vi "Create Log File.vi"(8 "error in":errorcluster, 11 "Sys Log in":refnum<class "System Log.lvclass">) -> (0 "error out":errorcluster, 3 "Sys Log out":refnum<class "System Log.lvclass">)   [LabVIEW 2014, in "System Log.lvclass"]
uses:
  System Log.lvclass
  System Log.lvclass/System Log.ctl
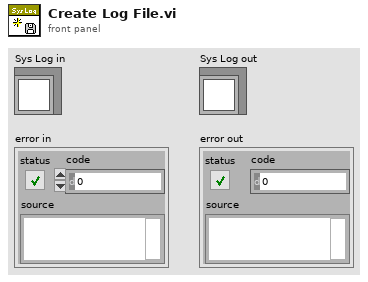
[diagram p1: front panel]
types:
  T1 = enum16{"open", "replace", "create", "open or create", "replace or create", "replace or create with confirmation"}
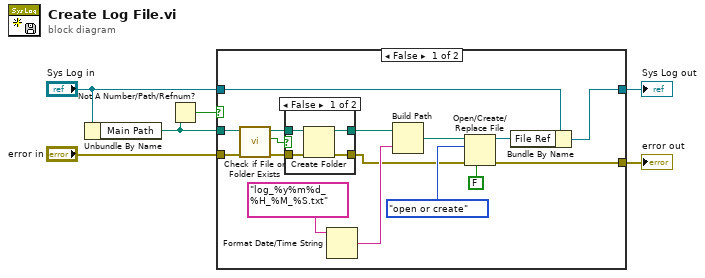
[diagram p0: block diagram]
diagram:
  n1 = Unbundle By Name("Sys Log in") -> ("Main Path"=w6:path)
  n2 = Not A Number/Path/Refnum?(number/path/refnum=w6) -> (NaN/Path/Refnum?=w1:bool)
  n3 = case shown="False" w1 {
    tunnel: "Sys Log in" -> [w22 w30]
    tunnel: [w21 w30] -> w3
    tunnel: "error in" -> [w15 w29]
    tunnel: [w19 w29] -> w5
    tunnel: w6 -> [w16 _]
    frame False {
      n4 = call <vilib>:"Check if File or Folder Exists.vi"("error in (no error)"=w15, "path"=w16) -> ("error out"=w12:errorcluster, "file or folder exists?"=w14:bool, "dup path"=w13:path)  [unwired: 7 in]
      n5 = case shown="False" w14 {
        tunnel: w13 -> [w26 w28]
        tunnel: w12 -> [w25 w27]
        tunnel: [w24 w28] -> w11
        tunnel: [w23 w27] -> w8
        frame False {
          n6 = Create Folder(path (use dialog)=w26, error in=w25) -> (created path=w24:path, error out=w23:errorcluster)  [unwired: 1 in, 1 out]
        }
        frame True {
        }
      }
      n7 = Format Date/Time String(time format string (%c)="log_%y%m%d_%H_%M_%S.txt") -> (date/time string=w10:string)  [unwired: 2 in]
      n8 = Build Path(base path=w11, name or relative path=w10) -> (appended path=w9:path)
      n9 = Open/Create/Replace File(file path (use dialog)=w9, error in=w8, operation (0:open)=T1."open or create", disable buffering (F)=FALSE) -> (refnum out=w20:refnum<file>, error out=w19:errorcluster)  [unwired: 2 in, 1 out]
      n10 = Bundle By Name(cluster=w22, "File Ref"=w20) -> (w21:refnum<class "System Log.lvclass">)
    }
    frame True {
    }
  }
  "error out" <- w5
  "Sys Log out" <- w3
